vi "PQsendQuery.vi"(8 "error in (no error)":errorcluster, 10 "query":string, 11 "conn":u64) -> (0 "error out":errorcluster, 2 "PQsendQuery":i64, 3 "conn_out":u64)   [LabVIEW 2019, in "libpqlv64.lvlib"]
doc: "Submits a command to the server without waiting for the result(s). 1 is returned if the command was successfully dispatched and 0 if not (in which case, use PQerrorMessage to get more information about the failure).\n\n int PQsendQuery(PGconn *conn, const char *command);\nhttp://www.postgresql.org/docs/8.3/static/libpq-async.html"
uses:
  libpqlv64.lvlib
  libpq.dll
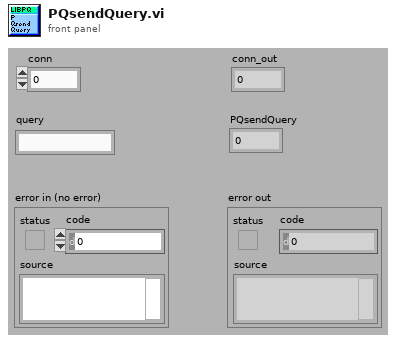
[diagram p1: front panel]
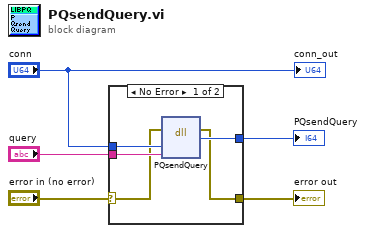
[diagram p0: block diagram]
diagram:
  n1 = case shown="No Error" "error in (no error)" {
    selector: "error in (no error)" -> [w7 w11]
    tunnel: [w6 w11] -> w4
    tunnel: [w10 _] -> w3
    tunnel: "query" -> [w9 _]
    tunnel: "conn" -> [w8 _]
    frame No Error {
      n2 = dll-call lib="libpq.*" fn="PQsendQuery"(error in=w7, "conn"=w8, "query"=w9) -> (error out=w6:errorcluster, "PQsendQuery"=w10:i64)  [unwired: 4 in, 1 out]
    }
    frame Error {
    }
  }
  "PQsendQuery" <- w3
  "error out" <- w4
  "conn_out" <- "conn"
